vi "Init Events.vi"(8 "error in (no error)":errorcluster, 11 "DiscoveryService in":refnum<class "DiscoveryService.lvclass">) -> (0 "error out":errorcluster, 3 "DiscoveryService out":refnum<class "DiscoveryService.lvclass">)   [LabVIEW 2020, in "Vecto.lvlib" / "DiscoveryService.lvclass"]
uses:
  DiscoveryService.lvclass
  Incoming Events.ctl
  Update Service Data.ctl
  lv-volatus/messages/Service/Data.ctl
  lv-volatus/messages/ServiceType/Enumeration.ctl
  Capabilities Update Data.ctl
  Capabilities Action.ctl
  DiscoveryService.lvclass/DiscoveryService.ctl
  lv-volatus/messages/ServiceType/ServiceType.lvlib
  lv-volatus/messages/Service/Service.lvlib
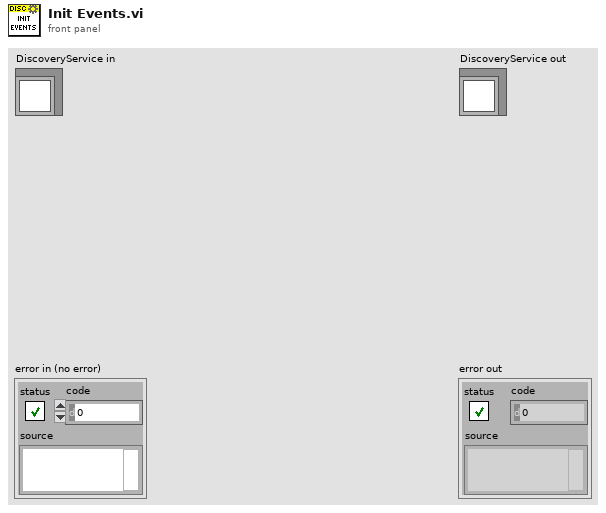
[diagram p1: front panel]
types:
  T1 = typedef "Vecto.lvlib/DiscoveryService.lvclass/Capabilities Update Data.ctl" = cluster{"Action":T2, "Capabilities":string[]}
  T2 = typedef "Vecto.lvlib/DiscoveryService.lvclass/Capabilities Action.ctl" = enum16{"Add", "Remove", "Clear"}
  T3 = typedef "ServiceType.lvlib/Enumeration.ctl" = enum16{"SERVICETYPE_UNKNOWN", "SERVICETYPE_TCPSERVER", "SERVICETYPE_HTTPSERVER"}
  T4 = typedef "Vecto.lvlib/DiscoveryService.lvclass/Update Service Data.ctl" = cluster{"Service":T5}
  T5 = typedef "Service.lvlib/Data.ctl" = cluster{"type":T3, "port":i32}
  T6 = typedef "Vecto.lvlib/DiscoveryService.lvclass/Incoming Events.ctl" = cluster{"Close":refnum<user-event>, "Update Service":refnum<user-event>, "Update Status":refnum<user-event>, "Remove Service":refnum<user-event>, "Update Cfg Version":refnum<user-event>, "Update Capabilities":refnum<user-event>}
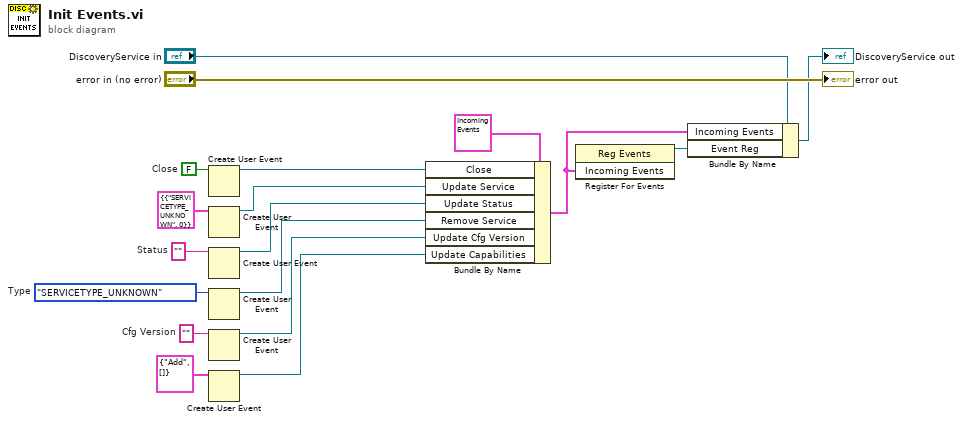
[diagram p0: block diagram]
diagram:
  w4 = ""  # Cfg Version
  w6 = Enumeration."SERVICETYPE_UNKNOWN"  # Type
  w8 = ""  # Status
  w17 = FALSE  # Close
  n1 = Create User Event(user event datatype=w17) -> (user event=w15:refnum<user-event>)  [unwired: 1 in, 1 out]
  n2 = Create User Event(user event datatype=T4 {"Service"={"type"=enum."SERVICETYPE_UNKNOWN", "port"=0}} ("Update Service Data")) -> (user event=w9:refnum<user-event>)  [unwired: 1 in, 1 out]
  n3 = Create User Event(user event datatype=w8) -> (user event=w7:refnum<user-event>)  [unwired: 1 in, 1 out]
  n4 = Create User Event(user event datatype=w6) -> (user event=w5:refnum<user-event>)  [unwired: 1 in, 1 out]
  n5 = Create User Event(user event datatype=w4) -> (user event=w3:refnum<user-event>)  [unwired: 1 in, 1 out]
  n6 = Create User Event(user event datatype=T1 {"Action"=enum."Add", "Capabilities"=[]} ("Capabilities Update Data")) -> (user event=w1:refnum<user-event>)  [unwired: 1 in, 1 out]
  n7 = Bundle By Name(cluster=T6 {"Close"=refnum, "Update Service"=refnum, "Update Status"=refnum, "Remove Service"=refnum, "Update Cfg Version"=refnum, "Update Capabilities"=refnum} ("Incoming Events"), "Close"=w15, "Update Service"=w9, "Update Status"=w7, "Remove Service"=w5, "Update Cfg Version"=w3, "Update Capabilities"=w1) -> (w13:T6)
  n8 = register-events(w13) -> (reference out=w12:refnum<event-registration>)  [unwired: 2 in, 1 out]
  n9 = Bundle By Name(cluster="DiscoveryService in", "Incoming Events"=w13, "Event Reg"=w12) -> (→"DiscoveryService out":refnum<class "DiscoveryService.lvclass">)
  "error out" <- "error in (no error)"
